vi "serial.vi"(6 "error in (no error)":errorcluster, 8 "Numeric":i32=30, 9 "Serial Port":refnum<visa-resource-name>) -> (0 "error out":errorcluster, 2 "Value":i16)   [LabVIEW 2018]
uses:
  <vilib>/Utility/error.llb/DialogType.ctl
  <vilib>/Instr/_visa.llb/VISA Configure Serial Port (Instr).vi
panel:
  out "unsigned byte array":u8[](array[numeric])
  out "substring":string
  out "Command":string
  out "read buffer":string
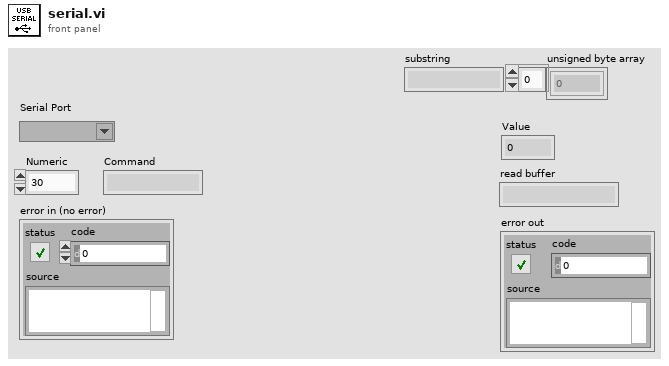
[diagram p1: front panel]
types:
  T1 = typedef "DialogType.ctl" = u16
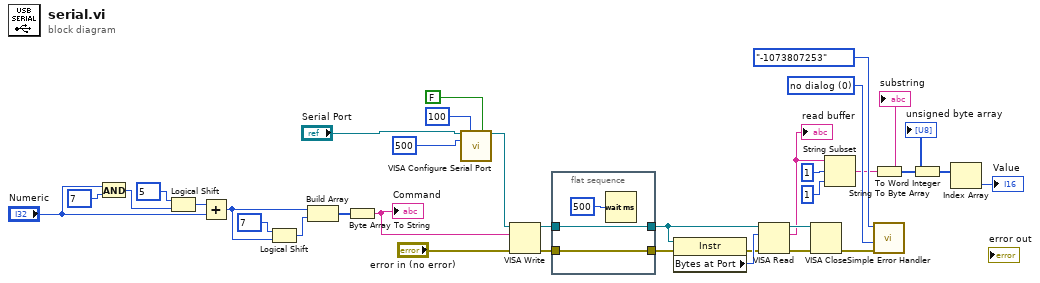
[diagram p0: block diagram]
diagram:
  w26 = T1 0 items=["no dialog", "OK message", "continue or stop message", "OK message + warnings", "continue/stop + warnings"] ("type of dialog (OK msg:1)")
  n1 = And(x="Numeric", y=7 ("0x7")) -> (x .and. y?=w6:i32)
  n2 = Logical Shift(y=5 ("x"), x=w6) -> (x << y=w9:i32)
  n3 = Add(x=w9, y="Numeric") -> (x+y=w2:i32)
  n4 = Logical Shift(y=i16 7, x=w2) -> (x << y=w3:i32)
  n5 = Build Array(w2, w3) -> (w4:i32[])
  n6 = Byte Array To String(unsigned byte array=w4) -> (string=w5:string)
  "Command" <- w5
  n7 = call-poly "VISA Configure Serial Port"("VISA resource name"="Serial Port", "timeout (10sec)"=u32 100, "Enable Termination\nChar (T)"=FALSE ("Enable Termination\nChar (T)"), "baud rate (9600)"=u32 500) -> ("VISA resource name out"=w32:refnum<visa-resource-name>)  [unwired: 10 in, 1 out]
  n8 = VISA Write(VISA resource name=w32, write buffer=w5, error in (no error)="error in (no error)") -> (VISA resource name out=w29:refnum<visa-resource-name>, error out=w21:errorcluster)  [unwired: 1 out]
  n9 = flat-sequence {
    tunnel: [w37] -> w28
    tunnel: w29 -> [w37]
    tunnel: [w35] -> w22
    tunnel: w21 -> [w35]
    frame #0 {
      n10 = Wait (ms)(milliseconds to wait=u32 500) -> ()  [unwired: 1 out]
    }
  }
  n11 = property class="Instr"(reference=w28, error in=w22) -> (error out=w20:errorcluster, "Bytes at Port"=w25:u32)  [unwired: 1 out]
  n12 = VISA Read(VISA resource name=w28, byte count=w25, error in (no error)=w20) -> (VISA resource name out=w16:refnum<visa-resource-name>, read buffer=w13:string, error out=w23:errorcluster)  [unwired: 1 out]
  "read buffer" <- w13
  n13 = VISA Close(VISA resource name=w16, error in (no error)=w23) -> (error out=w19:errorcluster)
  n14 = String Subset(string=w13, offset (0)=1, length (rest)=1 ("length (rest)")) -> (substring=w14:string)
  "substring" <- w14
  n15 = String To Byte Array(string=w14) -> (unsigned byte array=w15:u8[])
  "unsigned byte array" <- w15
  n16 = call <vilib>:"Simple Error Handler.vi"("error code (no error:0)"=enum16{"-1073807253"}."-1073807253", "type of dialog (OK msg:1)"=w26, "error in (no error)"=w19) -> ()  [unwired: 2 in, 5 out]
  n17 = To Word Integer(number=w15) -> (16bit integer=w12:i16[])
  n18 = Index Array(array=w12) -> (element=→"Value":i16)  [unwired: 1 in]
